vi "USB_CAN_Sync.vi"(1 "销毁":bool) -> (0 "Send Sync":T1)   [LabVIEW 2011]
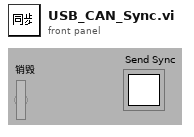
[diagram p1: front panel]
types:
  T1 = typedef "Rendezvous RefNum" = refnum<k1>
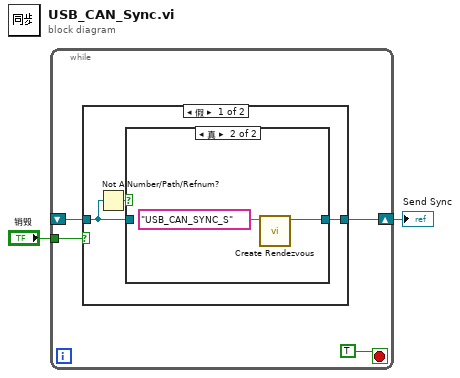
[diagram p0: block diagram]
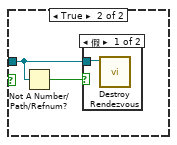
[diagram p3: hidden frame]
diagram:
  n1 = while {
    shift-right: [w4] -> w1
    shift-left: _ -> [w5]
    tunnel: "销毁" -> [w3]
    stop <- TRUE stop-if-true
    n2 = case shown="假" w3 {
      tunnel: w5 -> [w8 w13]
      tunnel: [w7 _] -> w4
      frame False {
        n3 = Not A Number/Path/Refnum?(number/path/refnum=w8) -> (NaN/Path/Refnum?=w9:bool)
        n4 = case shown="真" w9 {
          tunnel: w8 -> [w10 _]
          tunnel: [w10 w11] -> w7
          frame False {
          }
          frame True {
            n5 = call <vilib>:"Create Rendezvous.vi"("name (unnamed)"="USB_CAN_SYNC_S") -> ("rendezvous"=w11:T1)  [unwired: 4 in, 2 out]
          }
        }
      }
      frame True {
        n6 = Not A Number/Path/Refnum?(number/path/refnum=w13) -> (NaN/Path/Refnum?=w14:bool)
        n7 = case shown="假" w14 {
          tunnel: w13 -> [w15 _]
          frame False {
            n8 = call <vilib>:"Destroy Rendezvous.vi"("rendezvous"=w15) -> ()  [unwired: 5 in, 2 out]
          }
          frame True {
          }
        }
      }
    }
  }
  "Send Sync" <- w1
